vi "set_exp_to_groupSD.vi"(0 "Experiments groups":refnum<class "Experiments_group.lvclass">[](array[class]), 1 "exp selected":i32, 2 "group":u16, 3 "error in (no error)":errorcluster, 4 "New":bool, 5 "Experiment in":refnum<class "Experiment.lvclass">) -> (6 "Experiments groups out":refnum<class "Experiments_group.lvclass">[](array[class]), 7 "error out":errorcluster)   [LabVIEW 2015]
uses:
  Classes/Experiment.lvclass
  Classes/Experiments_group.lvclass
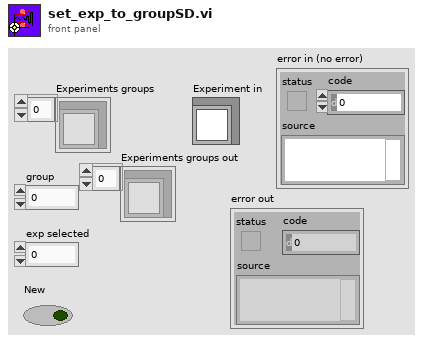
[diagram p1: front panel]
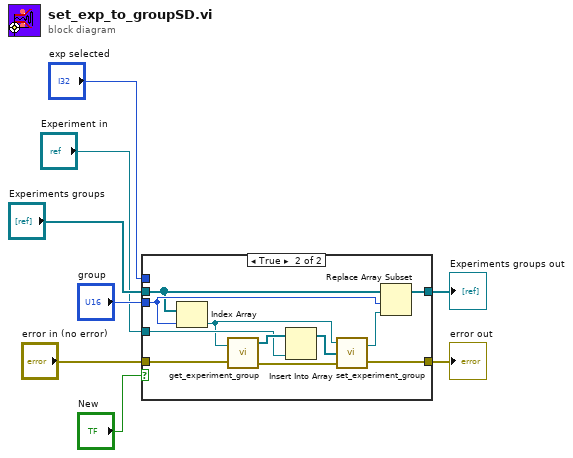
[diagram p0: block diagram]
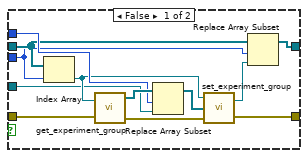
[diagram p2: hidden frame]
diagram:
  n1 = case shown="True" "New" {
    tunnel: "error in (no error)" -> [w20 w31]
    tunnel: "exp selected" -> [w18 _]
    tunnel: "Experiments groups" -> [w14 w24]
    tunnel: "group" -> [w13 w25]
    tunnel: [w12 w23] -> w4
    tunnel: [w10 w22] -> w3
    tunnel: "Experiment in" -> [w9 w29]
    frame False {
      n2 = Index Array(array=w14, index=w13) -> (element=w16:refnum<class "Experiments_group.lvclass">)
      n3 = call-dynamic "get_experiment_group.vi"("Experiments_group.lvclass in"=w16, "error in (no error)"=w20) -> ("Experiments"=w19:refnum<class "Experiment.lvclass">[], "error out"=w11:errorcluster)  [unwired: 1 out]
      n4 = Replace Array Subset(array=w19, new element=w9, index=w18) -> (w17:refnum<class "Experiment.lvclass">[])
      n5 = call-dynamic "set_experiment_group.vi"("error in (no error)"=w11, "Experiments"=w17, "Experiments_group.lvclass in"=w16) -> ("error out"=w10:errorcluster, "Experiments_group.lvclass out"=w15:refnum<class "Experiments_group.lvclass">)
      n6 = Replace Array Subset(array=w14, new element=w15, index=w13) -> (w12:refnum<class "Experiments_group.lvclass">[])
    }
    frame True {
      n7 = Index Array(array=w24, index=w25) -> (element=w27:refnum<class "Experiments_group.lvclass">)
      n8 = call-dynamic "get_experiment_group.vi"("Experiments_group.lvclass in"=w27, "error in (no error)"=w31) -> ("Experiments"=w30:refnum<class "Experiment.lvclass">[], "error out"=w21:errorcluster)  [unwired: 1 out]
      n9 = Insert Into Array(array=w30, new element=w29) -> (w28:refnum<class "Experiment.lvclass">[])  [unwired: 1 in]
      n10 = call-dynamic "set_experiment_group.vi"("error in (no error)"=w21, "Experiments"=w28, "Experiments_group.lvclass in"=w27) -> ("error out"=w22:errorcluster, "Experiments_group.lvclass out"=w26:refnum<class "Experiments_group.lvclass">)
      n11 = Replace Array Subset(array=w24, new element=w26, index=w25) -> (w23:refnum<class "Experiments_group.lvclass">[])
    }
  }
  "error out" <- w3
  "Experiments groups out" <- w4
